vi "Query Conditions.vi"() -> ()   [LabVIEW 2024]
uses:
  <vilib>/Plug-In SDKs/Clients/Data Store V1/Data Store Client.lvlibp
  <vilib>/Plug-In SDKs/Clients/Data Store V1/Data Store Client.lvlibp/API/Data Store V1/Read Condition Value (Double Array).vi
panel:
  in  "odata query":string="$filter=contains(Name,'Temperature') or contains(Name,'Pressure')"
  out "queried conditions":T1(array[cluster])
  out "error out":errorcluster
  # "Query Conditions\n\nThis example shows you to use odata to query for published conditions.\nRun Publish Data.vi to create the data that is queried by this VI."
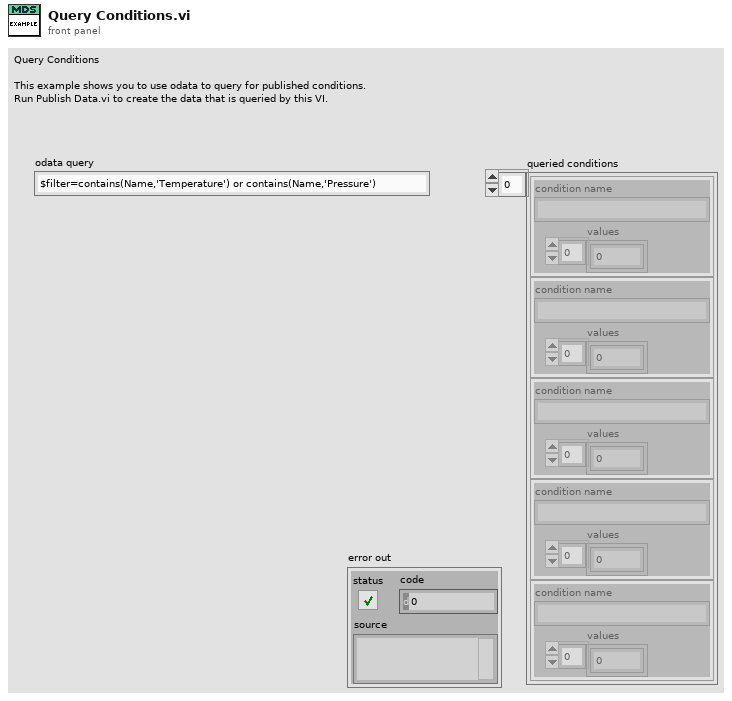
[diagram p1: front panel]
types:
  T1 = cluster{"condition name":string, "values":dbl[]}[]
  T2 = typedef "Data Store Client.lvlibp/Published Condition.ctl" = cluster{"name":string, "condition type":string, "moniker":T3, "id":string, "step id":string, "test result id":string}
  T3 = typedef "Data Store Client.lvlibp/Data Moniker.ctl" = cluster{"service location":string, "data source":string, "data instance":i64}
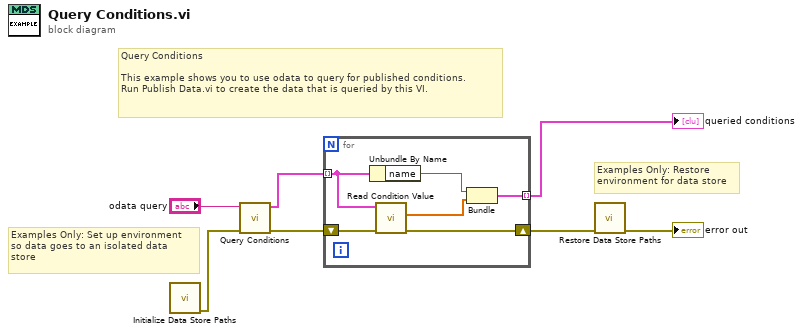
[diagram p0: block diagram]
diagram:
  # "Examples Only: Restore\nenvironment for data store"
  # "Examples Only: Set up environment\nso data goes to an isolated data\nstore"
  # "Query Conditions\n\nThis example shows you to use odata to query for published conditions.\nRun Publish Data.vi to create the data that is queried by this VI."
  n1 = call "Initialize Data Store Paths.vi"() -> ("error out"=w3:errorcluster)  [unwired: 11 in]
  n2 = call <vilib>:"Query Conditions.vi"("error in"=w3, "odata query"="odata query") -> ("error out"=w6:errorcluster, "published conditions"=w4:T2[])  [unwired: 8 in]
  n3 = for {
    tunnel: w4 -> [w8] mode=indexing
    shift-right: [w11] -> w2
    shift-left: w6 -> [w10]
    tunnel: [w12] -> w5 mode=indexing
    n4 = Unbundle By Name(w8) -> ("name"=w13:string)
    n5 = call-poly <vilib>:"Read Condition Value.vi"("error in"=w10, "published condition"=w8) -> ("error out"=w11:errorcluster, "values"=w9:dbl[])  [unwired: 6 in, 2 out]
    n6 = Bundle("name"=w13, "values"=w9) -> (w12:cluster{"name":string, "values":dbl[]})  [unwired: 1 in]
  }
  "queried conditions" <- w5
  n7 = call "Restore Data Store Paths.vi"("error in"=w2) -> ("error out"=→"error out":errorcluster)  [unwired: 10 in]
